vi "Write File.vi"(8 "error in (no error)":errorcluster, 9 "Data":variant, 10 "datalog path (use dialog)":path, 11 "File Interface in":refnum<class "File Interface.lvclass">) -> (0 "error out":errorcluster)   [LabVIEW 2018, in "ImportExport.lvlib" / "File Interface.lvclass"]
uses:
  Switch Configuration.llb/File Interface.lvclass
  Switch Configuration.llb/SysDef.Globals.vi
  Switch Configuration.llb/Advanced System Definition.lvlib
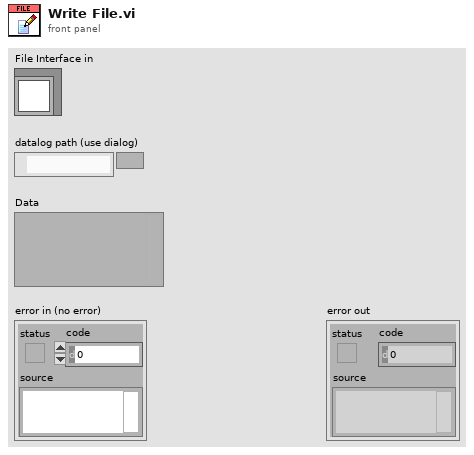
[diagram p1: front panel]
types:
  T1 = enum16{"open", "replace", "create", "open or create", "replace or create", "replace or create with confirmation"}
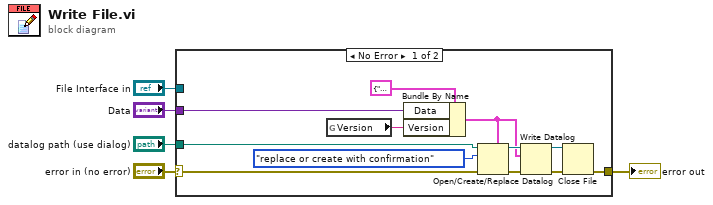
[diagram p0: block diagram]
diagram:
  n1 = case shown="No Error" "error in (no error)" {
    selector: "error in (no error)" -> [w9 w18]
    tunnel: [w8 w18] -> w4
    tunnel: "File Interface in" -> [_ _]
    tunnel: "Data" -> [w10 _]
    tunnel: "datalog path (use dialog)" -> [w7 _]
    frame No Error {
      n2 = global read "SysDef.Globals.vi" "Version"() -> (w6:string)
      n3 = Bundle By Name(cluster=cluster{"Version":string, "Data":variant} {"Version"="", "Data"=variant}, "Data"=w10, "Version"=w6) -> (w13:cluster{"Version":string, "Data":variant})
      n4 = Open/Create/Replace Datalog(5:w13, 8:w9, 10:T1."replace or create with confirmation" ("operation (0:open)"), 11:w7) -> (0:w15:errorcluster, 3:w14:refnum<k1>)  [unwired: 2 in, 1 out]
      n5 = Write Datalog(4:w15, 6:w13, 7:w14) -> (0:w12:errorcluster, 3:w11:refnum<k1>)
      n6 = Close File(refnum=w11, error in=w12) -> (error out=w8:errorcluster)  [unwired: 1 out]
    }
    frame Error {
    }
  }
  "error out" <- w4
